vi "U6 Single AIN noise testing.vi"() -> (0 "error out":errorcluster)   [LabVIEW 2021]
panel:
  out "ENOB (RMS)":dbl format="%.2f"
  out "ENOB (max-min)":dbl format="%.2f"
  out "Time Per Iteration (ms)":dbl format="%.2f"
  out "Time (ms)":u32
  in  "Negative Channel #":i32=199
  out "Max-Min":dbl format="%.9f"
  out "SD":dbl format="%.9f"
  out "Max":dbl format="%.9f"
  out "Min":dbl format="%.9f"
  in  "Iterations":i32=128
  in  "AIN Range":u16(ring) items=["LJ_rgBIP10V", "LJ_rgBIP1V", "LJ_rgBIPP1V", "LJ_rgBIPP01V"]
  in  "Binary":bool
  in  "SettlingFactor":i32
  in  "Resolution":i32=1
  in  "FirstFound":bool=TRUE
  in  "Address":string="1"
  out "Error Message":string
  out "Avg Value Read":dbl format="%.9f"
  in  "Positive Channel #":i32=15
  # "Configures and reads 1 analog input."
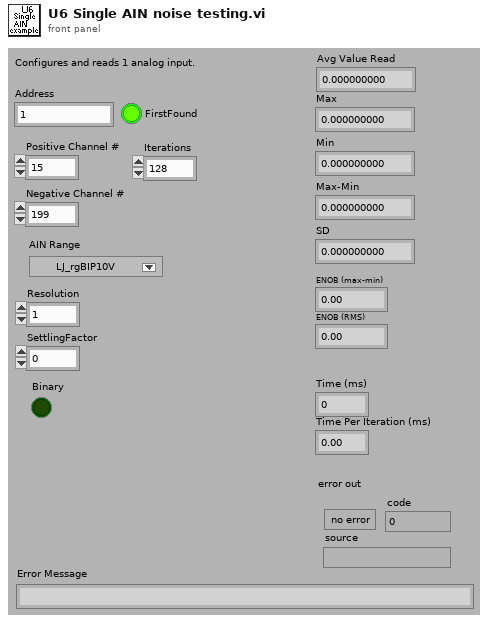
[diagram p1: front panel]
types:
  T1 = cluster{"Avg":dbl, "Std Dev (RMS)":dbl, "Max":dbl, "Min":dbl, "max-min":dbl}
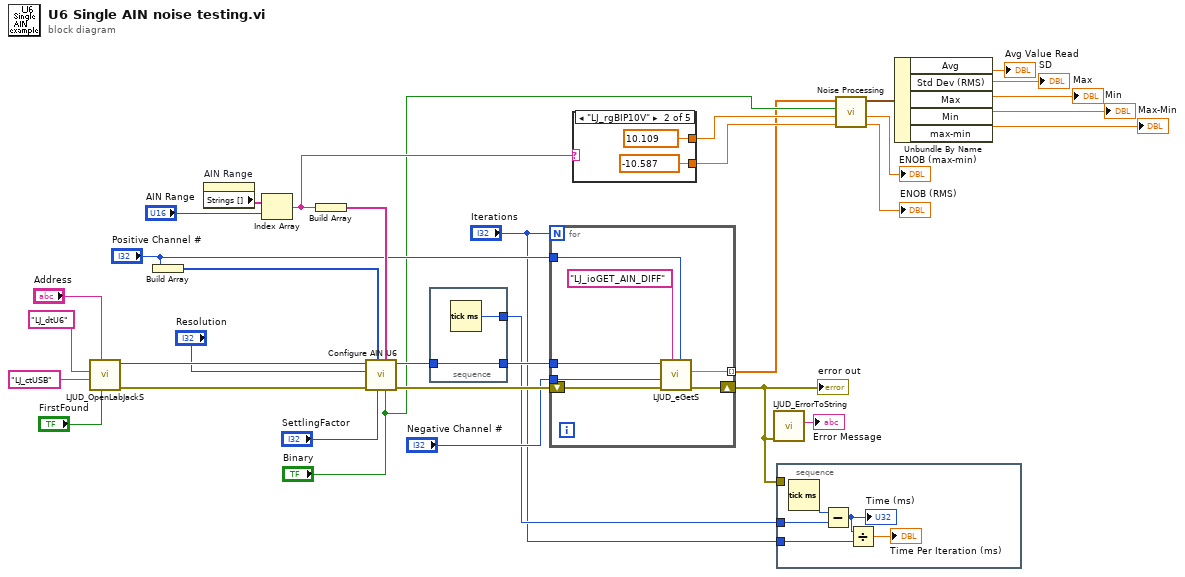
[diagram p0: block diagram]
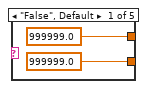
[diagram p2: hidden frame]
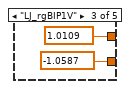
[diagram p3: hidden frame]
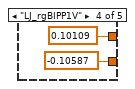
[diagram p4: hidden frame]
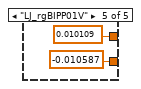
[diagram p5: hidden frame]
diagram:
  n1 = call "LJUD_OpenLabJackS.vi"("FirstFound"="FirstFound", "Address"="Address", "ConnectionType"="LJ_ctUSB", "DeviceType"="LJ_dtU6") -> ("error out"=w28:errorcluster, "Handle"=w29:i32)  [unwired: 5 in, 1 out]
  n2 = Build Array("Positive Channel #") -> (w25:i32[])
  n3 = property on="AIN Range" class="Ring (strict)"() -> ("Strings []"=w27:string[])  [unwired: 2 in, 2 out]
  n4 = Index Array(array=w27, index="AIN Range") -> (element=w13:string)
  n5 = Build Array(w13) -> (w24:string[])
  n6 = call "Configure AIN U6.vi"("Binary"="Binary", "Ranges"=w24, "SettlingFactor"="SettlingFactor", "Positive Channels"=w25, "error in"=w28, "Resolution"="Resolution", "Handle In"=w29) -> ("error out"=w21:errorcluster, "Handle Out"=w18:i32)  [unwired: 3 in]
  n7 = stacked-sequence {
    tunnel: w18 -> [w36]
    tunnel: [w36] -> w17
    tunnel: [w35] -> w15
    frame #0 {
      n8 = Tick Count (ms)() -> (millisecond timer value=w35:u32)
    }
  }
  n9 = for {
    N: "Iterations" -> [_]
    tunnel: [w43] -> w9 mode=indexing
    tunnel: w17 -> [w41]
    tunnel: "Positive Channel #" -> [w40]
    tunnel: "Negative Channel #" -> [w39]
    shift-right: [w37] -> w16
    shift-left: w21 -> [w38]
    n10 = call "LJUD_eGetS.vi"("Channel"=w40, "IOType"="LJ_ioGET_AIN_DIFF", "error in"=w38, "x1"=w39, "Handle In"=w41) -> ("error out"=w37:errorcluster, "Value Read"=w43:dbl)  [unwired: 4 in, 1 out]
  }
  "error out" <- w16
  n11 = case shown="\"LJ_rgBIP10V\"" w13 {
    tunnel: [999999.0 10.109 1.0109 0.10109 0.010109] -> w12
    tunnel: [999999.0 -10.587 -1.0587 -0.10587 -0.010587] -> w11
    frame "False", Default {
    }
    frame "LJ_rgBIP10V" {
    }
    frame "LJ_rgBIP1V" {
    }
    frame "LJ_rgBIPP1V" {
    }
    frame "LJ_rgBIPP01V" {
    }
  }
  n12 = call "LJUD_ErrorToString.vi"("error in"=w16) -> ("String"=→"Error Message":string)  [unwired: 10 in]
  n13 = stacked-sequence {
    tunnel: w16 -> [_]
    tunnel: w15 -> [w57]
    tunnel: "Iterations" -> [w55]
    frame #0 {
      n14 = Tick Count (ms)() -> (millisecond timer value=w58:u32)
      n15 = Subtract(x=w58, y=w57) -> (x-y=w56:u32)
      "Time (ms)" <- w56
      n16 = Divide(x=w56, y=w55) -> (x/y=→"Time Per Iteration (ms)":dbl)
    }
  }
  n17 = call "Noise Processing.vi"("Min Voltage"=w11, "Max Voltage"=w12, "16-bit Binary"="Binary", "Data"=w9) -> ("ENOB (RMS)"=→"ENOB (RMS)":dbl, "ENOB (max-min)"=→"ENOB (max-min)":dbl, "Results"=w8:T1)  [unwired: 3 in, 2 out]
  n18 = Unbundle By Name(w8) -> ("Avg"=→"Avg Value Read":dbl, "Std Dev (RMS)"=→"SD":dbl, "Max"=→"Max":dbl, "Min"=→"Min":dbl, "max-min"=→"Max-Min":dbl)
